vi "LVProjectShortcut_RegisterOverlays.vi"(8 "error in":errorcluster, 11 "Item":T1) -> (0 "error out":errorcluster)   [LabVIEW 2017]
doc: "Registers a set of Icon Overlay Aliases and tells the framework where to find the .ico files matching\nthese Aliases."
uses:
  <resource>/Framework/Providers/API/ItemRef.ctl
  <resource>/Framework/Providers/API/mxLvOverlayAlias.ctl
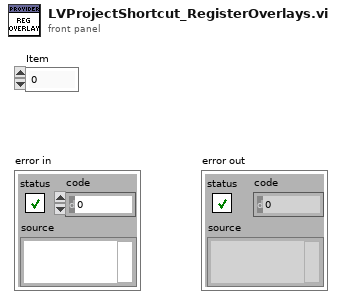
[diagram p1: front panel]
types:
  T1 = typedef "ItemRef.ctl" = u64
  T2 = typedef "mxLvOverlayAlias.ctl" = cluster{"Overlay Alias":string, "Icon File Name":path}
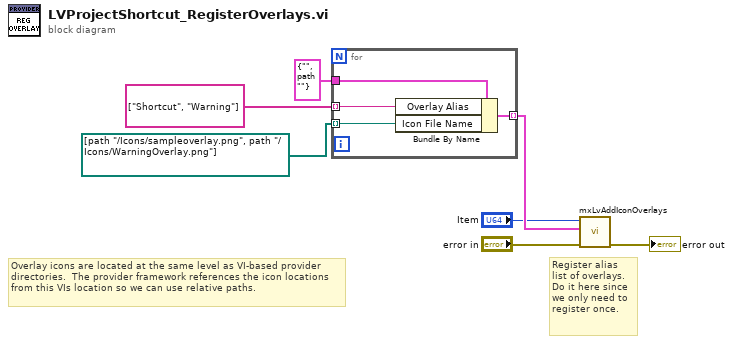
[diagram p0: block diagram]
diagram:
  # "Overlay icons are located at the same level as VI-based provider directories.  The provider framework references the icon locations from this VIs location so we can use relative paths."
  # "Register alias list of overlays.  Do it here since we only need to register once."
  n1 = for {
    tunnel: T2 {"Overlay Alias"="", "Icon File Name"=path ""} ("Icon Overlay Alias") -> [w11]
    tunnel: [w10] -> w7 mode=indexing
    tunnel: string[] ["Shortcut", "Warning"] ("overlay alias") -> [w9] mode=indexing
    tunnel: path[] [path "../Icons/sampleoverlay.png", path "../Icons/WarningOverlay.png"] ("icon filename") -> [w8] mode=indexing
    n2 = Bundle By Name(cluster=w11, "Overlay Alias"=w9, "Icon File Name"=w8) -> (w10:T2)
  }
  n3 = call <resource>:"mxLvAddIconOverlays.vi"("error in"="error in", "Overlay Aliases"=w7, "Item"="Item") -> ("error out"=→"error out":errorcluster)  [unwired: 7 in, 1 out]
